vi "Get Child position from index Same Level.vi"(10 "TreeItem Index":i32, 11 "TreeItems":T1[](array[typedef])) -> (1 "Parent Tag Index":i32, 2 "Child Position":i32, 3 "Parent Tag":string)   [LabVIEW 2020, in "BetterDragAndDrop.lvlib" / "BetterTreeHandle.lvclass"]
uses:
  BetterTreeHandle/BetterTreeHandle.lvclass
  TreeItem.ctl
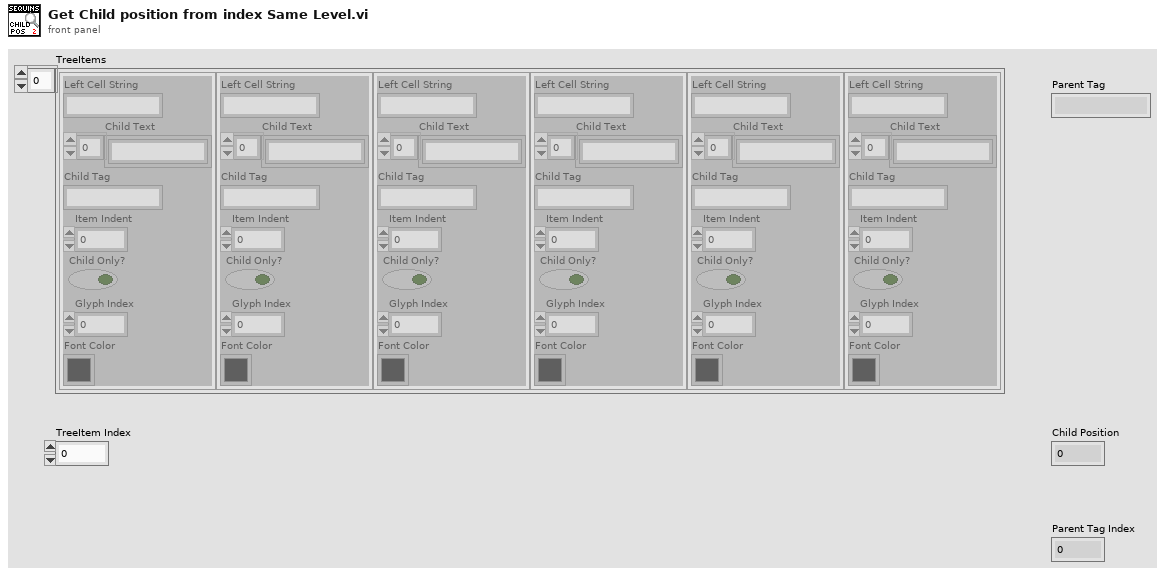
[diagram p1: front panel]
types:
  T1 = typedef "BetterDragAndDrop.lvlib/BetterTreeHandle.lvclass/TreeItem.ctl" = cluster{"Left Cell String":string, "Child Text":string[], "Child Tag":string, "Item Indent":i32, "Child Only?":bool, "Glyph Index":i32, "Font Color":u32}
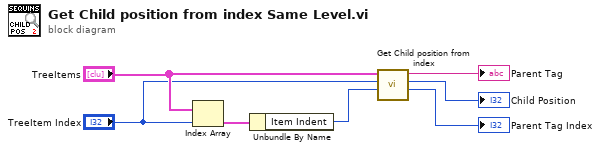
[diagram p0: block diagram]
diagram:
  n1 = Index Array(array="TreeItems", index="TreeItem Index") -> (element=w7:T1)
  n2 = Unbundle By Name(w7) -> ("Item Indent"=w5:i32)
  n3 = call "Get Child position from index.vi"("Insertion indent"=w5, "Insertion index"="TreeItem Index", "TreeItems (current)"="TreeItems") -> ("Parent Tag Index"=→"Parent Tag Index":i32, "Child Position"=→"Child Position":i32, "Parent Tag"=→"Parent Tag":string)  [unwired: 6 in]
